vi "Create Pattern Script - Rd Load Data Frame.vi"(8 "error in (no error)":errorcluster, 10 "Num of Cycles":i8, 11 "BML Pattern Creater in":refnum<class "BML Pattern Creater.lvclass">) -> (0 "error out":errorcluster, 2 "Rd Capture":string, 3 "BML Pattern Creater out":refnum<class "BML Pattern Creater.lvclass">)   [LabVIEW 2018, in "BML Pattern Creater.lvlib" / "BML Pattern Creater.lvclass"]
uses:
  BML Pattern Creater.lvclass
  Ctls/OM - BML.ctl
  BML Pattern Creater.lvclass/BML Pattern Creater.ctl
  Write BML OM.vi
  Read Frame Data.vi
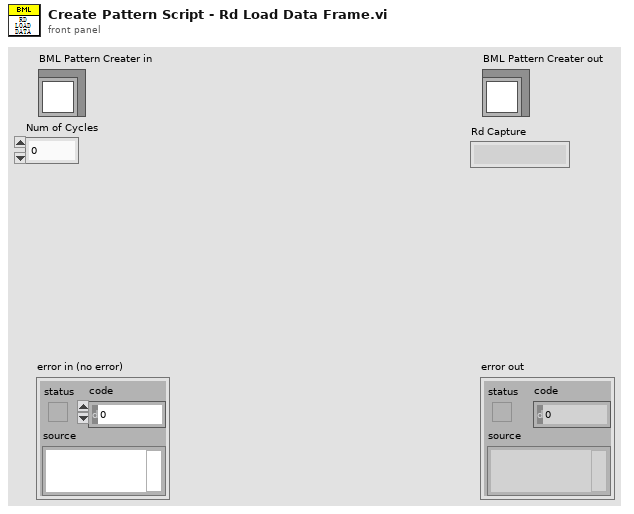
[diagram p1: front panel]
types:
  T1 = typedef "OM - BML.ctl" = enum16{"Normal", "ImmeEffect", "InitSlaveID", "LoadData"}
  T2 = typedef "FRM Data - BML.ctl" = cluster{"Pattern_Name":string, "Data":u8[], "Start_Addr":u16, "ChipID":u8, "num of wait ms":i8, "Opcode":string[], "BML OM":T1, "BurstLength":T3, "FSN":u8, "R/W?":T4}
  T3 = typedef "Burst Length.ctl" = enum8{"0", "2", "3", "4", "5", "8", "16", "32"}
  T4 = typedef "RW Options.ctl" = enum16{"Read", "Write", "R/W"}
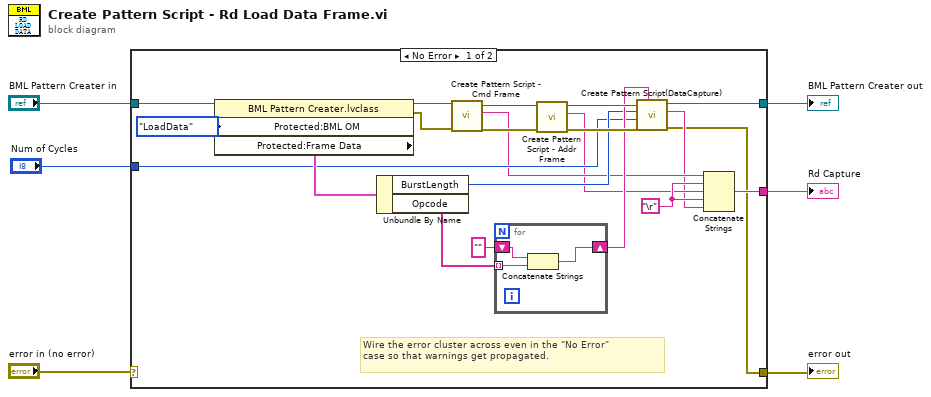
[diagram p0: block diagram]
diagram:
  # "Wire the error cluster across even in the \"No Error\"\ncase so that warnings get propagated."
  n1 = case shown="No Error" "error in (no error)" {
    selector: "error in (no error)" -> [_ w32]
    tunnel: [w7 w32] -> w1
    tunnel: "Num of Cycles" -> [w12 _]
    tunnel: [w24 _] -> w3
    tunnel: "BML Pattern Creater in" -> [w23 w31]
    tunnel: [w8 w31] -> w4
    frame No Error {
      w25 = "\r"
      n2 = property class="BML Pattern Creater.lvclass"(reference=w23, "Protected:BML OM"=OM_-_BML."LoadData" ("BML OM")) -> (reference out=w20:refnum<class "BML Pattern Creater.lvclass">, error out=w19:errorcluster, "Protected:Frame Data"=w21:T2)  [unwired: 1 in]
      n3 = Unbundle By Name(w21) -> ("BurstLength"=w13:T3, "Opcode"=w27:string[])
      n4 = call "Create Pattern Script - Cmd Frame.vi"("error in (no error)"=w19, "BML Pattern Creater in"=w20) -> ("error out"=w17:errorcluster, "CMD Frame out"=w11:string, "BML Pattern Creater out"=w18:refnum<class "BML Pattern Creater.lvclass">)  [unwired: 7 in]
      n5 = for {
        tunnel: w27 -> [w30] mode=indexing
        shift-right: [w29] -> w14
        shift-left: "" -> [w28]
        n6 = Concatenate Strings(w28, w30) -> (w29:string)
      }
      n7 = call "Create Pattern Script - Addr Frame.vi"("error in (no error)"=w17, "BML Pattern Creater in"=w18) -> ("error out"=w15:errorcluster, "Addr Frame"=w10:string, "BML Pattern Creater out"=w16:refnum<class "BML Pattern Creater.lvclass">)  [unwired: 7 in]
      n8 = call "Create Pattern Script(DataCapture).vi"("Opcode"=w14, "error in (no error)"=w15, "Num of Cycles"=w12, "BurstLength"=w13, "BML Pattern Creater in"=w16) -> ("error out"=w7:errorcluster, "String"=w9:string, "BML Pattern Creater out"=w8:refnum<class "BML Pattern Creater.lvclass">)  [unwired: 4 in]
      n9 = Concatenate Strings(w11, w25, w10, w25, w9) -> (w24:string)
    }
    frame Error {
    }
  }
  "error out" <- w1
  "BML Pattern Creater out" <- w4
  "Rd Capture" <- w3
